vi "open close simple table.vi"(8 "error in (no error)":errorcluster) -> (0 "error out":errorcluster)   [LabVIEW 2020]
uses:
  forms AF/Autoclose manager/Form ID.ctl
  forms AF/Open Close Logic Simple Table/Open Close Logic Simple Table.lvclass
  <vilib>/addons/_JKI Toolkits/Caraya/classes/Assert/Assert Equal Value_Variant.vi
  forms AF/Form Server Interfaces.lvlib
  <vilib>/addons/_JKI Toolkits/Caraya/classes/Assert/Assert.lvclass
  <vilib>/addons/_JKI Toolkits/Caraya/classes/Test/Test.lvclass
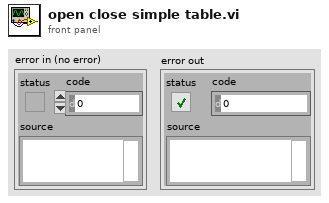
[diagram p1: front panel]
types:
  T1 = typedef "Form Server Interfaces.lvlib/Form ID.ctl" = cluster{"Name":string, "Panel type":string}
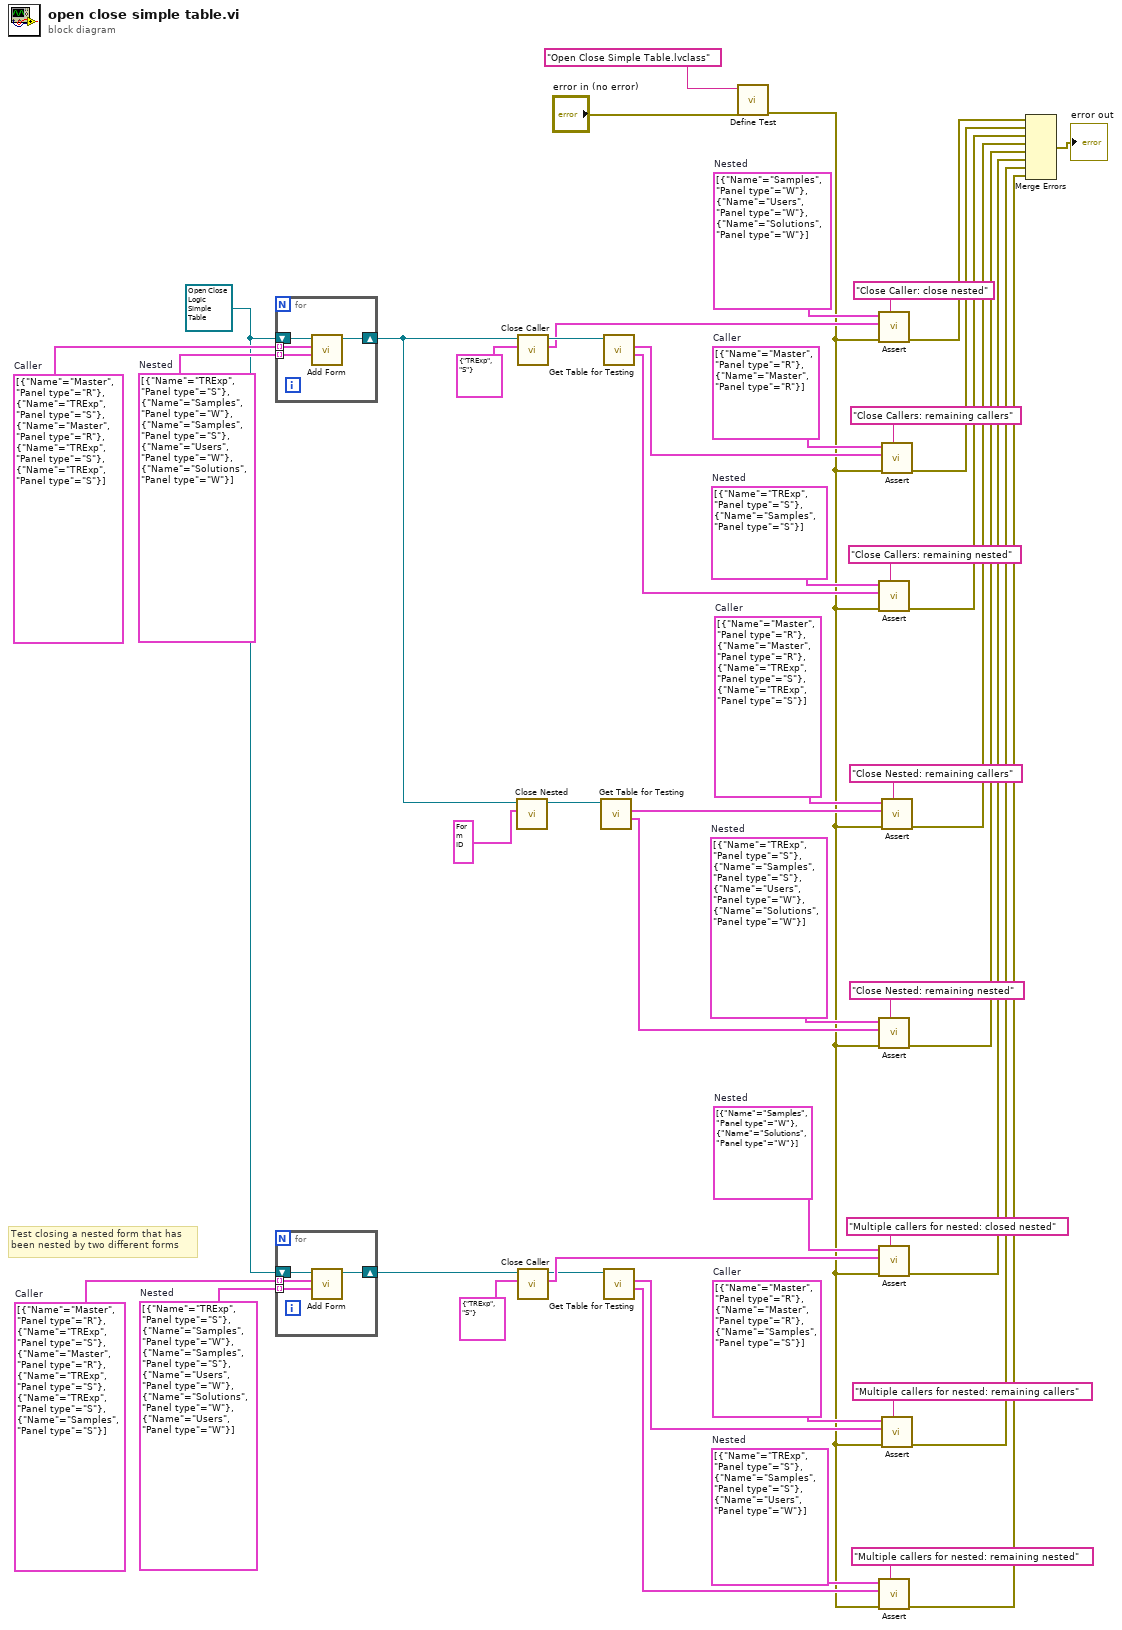
[diagram p0: block diagram]
diagram:
  w25 = T1[] [{"Name"="TRExp", "Panel type"="S"}, {"Name"="Samples", "Panel type"="S"}, {"Name"="Users", "Panel type"="W"}]  # Nested
  w21 = T1[] [{"Name"="Samples", "Panel type"="W"}, {"Name"="Solutions", "Panel type"="W"}]  # Nested
  w23 = T1[] [{"Name"="Master", "Panel type"="R"}, {"Name"="Master", "Panel type"="R"}, {"Name"="Samples", "Panel type"="S"}]  # Caller
  w31 = T1[] [{"Name"="TRExp", "Panel type"="S"}, {"Name"="Samples", "Panel type"="S"}, {"Name"="Users", "Panel type"="W"}, {"Name"="Solutions", "Panel type"="W"}]  # Nested
  w32 = T1[] [{"Name"="Master", "Panel type"="R"}, {"Name"="Master", "Panel type"="R"}, {"Name"="TRExp", "Panel type"="S"}, {"Name"="TRExp", "Panel type"="S"}]  # Caller
  w37 = T1[] [{"Name"="TRExp", "Panel type"="S"}, {"Name"="Samples", "Panel type"="S"}]  # Nested
  w41 = T1[] [{"Name"="Samples", "Panel type"="W"}, {"Name"="Users", "Panel type"="W"}, {"Name"="Solutions", "Panel type"="W"}]  # Nested
  w39 = T1[] [{"Name"="Master", "Panel type"="R"}, {"Name"="Master", "Panel type"="R"}]  # Caller
  w44 = T1[] [{"Name"="TRExp", "Panel type"="S"}, {"Name"="Samples", "Panel type"="W"}, {"Name"="Samples", "Panel type"="S"}, {"Name"="Users", "Panel type"="W"}, {"Name"="Solutions", "Panel type"="W"}, {"Name"="Users", "Panel type"="W"}]  # Nested
  w43 = T1[] [{"Name"="Master", "Panel type"="R"}, {"Name"="TRExp", "Panel type"="S"}, {"Name"="Master", "Panel type"="R"}, {"Name"="TRExp", "Panel type"="S"}, {"Name"="TRExp", "Panel type"="S"}, {"Name"="Samples", "Panel type"="S"}]  # Caller
  w26 = refnum<class "Open Close Logic Simple Table.lvclass"> refnum ("Open Close Logic Simple Table.lvlib:Open Close Logic Simple Table.lvclass")
  w48 = T1[] [{"Name"="TRExp", "Panel type"="S"}, {"Name"="Samples", "Panel type"="W"}, {"Name"="Samples", "Panel type"="S"}, {"Name"="Users", "Panel type"="W"}, {"Name"="Solutions", "Panel type"="W"}]  # Nested
  w49 = T1[] [{"Name"="Master", "Panel type"="R"}, {"Name"="TRExp", "Panel type"="S"}, {"Name"="Master", "Panel type"="R"}, {"Name"="TRExp", "Panel type"="S"}, {"Name"="TRExp", "Panel type"="S"}]  # Caller
  # "Test closing a nested form that has\nbeen nested by two different forms"
  n1 = for {
    tunnel: w49 -> [w51] mode=indexing
    tunnel: w48 -> [w50] mode=indexing
    shift-right: [w53] -> w47
    shift-left: w26 -> [w52]
    n2 = call-dynamic "Add Form.vi"("Nested"=w50, "Caller"=w51, "Autoclose manager in"=w52) -> ("Autoclose manager out"=w53:refnum<class "Open Close Logic Simple Table.lvclass">)  [unwired: 6 in, 2 out]
  }
  n3 = for {
    tunnel: w43 -> [w55] mode=indexing
    tunnel: w44 -> [w54] mode=indexing
    shift-right: [w57] -> w17
    shift-left: w26 -> [w56]
    n4 = call-dynamic "Add Form.vi"("Nested"=w54, "Caller"=w55, "Autoclose manager in"=w56) -> ("Autoclose manager out"=w57:refnum<class "Open Close Logic Simple Table.lvclass">)  [unwired: 6 in, 2 out]
  }
  n5 = call-dynamic "Close Nested.vi"("Nested"=T1 {"Name"="Samples", "Panel type"="W"}, "Open Close Logic Simple Table in"=w47) -> ("Open Close Logic Simple Table out"=w45:refnum<class "Open Close Logic Simple Table.lvclass">)  [unwired: 8 in, 1 out]
  n6 = call-dynamic "Close Caller.vi"("Caller"=T1 {"Name"="TRExp", "Panel type"="S"}, "Open Close Logic Simple Table in"=w47) -> ("Close Nested"=w42:T1[], "Open Close Logic Simple Table out"=w46:refnum<class "Open Close Logic Simple Table.lvclass">)  [unwired: 7 in, 1 out]
  n7 = call-dynamic "Close Caller.vi"("Caller"=T1 {"Name"="TRExp", "Panel type"="S"}, "Open Close Logic Simple Table in"=w17) -> ("Close Nested"=w20:T1[], "Open Close Logic Simple Table out"=w19:refnum<class "Open Close Logic Simple Table.lvclass">)  [unwired: 7 in, 1 out]
  n8 = call "Get Table for Testing.vi"("Open Close Logic Simple Table in"=w45) -> ("Nested"=w29:T1[], "Caller"=w30:T1[])  [unwired: 7 in, 2 out]
  n9 = call "Get Table for Testing.vi"("Open Close Logic Simple Table in"=w46) -> ("Nested"=w38:T1[], "Caller"=w40:T1[])  [unwired: 7 in, 2 out]
  n10 = call "Get Table for Testing.vi"("Open Close Logic Simple Table in"=w19) -> ("Nested"=w24:T1[], "Caller"=w22:T1[])  [unwired: 7 in, 2 out]
  n11 = call <vilib>:"Define Test.vi"("error in (no error)"="error in (no error)", "Label (VI Title)"="Open Close Simple Table.lvclass") -> ("error out"=w12:errorcluster)  [unwired: 9 in]
  n12 = call-poly <vilib>:"Assert.vi"("Label"="Close Caller: close nested", "error in (no error)"=w12, "Y"=w42, "X"=w41) -> ("error out"=w36:errorcluster)  [unwired: 7 in]
  n13 = call-poly <vilib>:"Assert.vi"("Label"="Close Callers: remaining nested", "error in (no error)"=w12, "Y"=w38, "X"=w37) -> ("error out"=w34:errorcluster)  [unwired: 7 in]
  n14 = call-poly <vilib>:"Assert.vi"("Label"="Close Nested: remaining nested", "error in (no error)"=w12, "Y"=w29, "X"=w31) -> ("error out"=w27:errorcluster)  [unwired: 7 in]
  n15 = call-poly <vilib>:"Assert.vi"("Label"="Multiple callers for nested: closed nested", "error in (no error)"=w12, "Y"=w20, "X"=w21) -> ("error out"=w15:errorcluster)  [unwired: 7 in]
  n16 = call-poly <vilib>:"Assert.vi"("Label"="Multiple callers for nested: remaining nested", "error in (no error)"=w12, "Y"=w24, "X"=w25) -> ("error out"=w7:errorcluster)  [unwired: 7 in]
  n17 = call-poly <vilib>:"Assert.vi"("Label"="Close Callers: remaining callers", "error in (no error)"=w12, "Y"=w40, "X"=w39) -> ("error out"=w35:errorcluster)  [unwired: 7 in]
  n18 = call-poly <vilib>:"Assert.vi"("Label"="Close Nested: remaining callers", "error in (no error)"=w12, "Y"=w30, "X"=w32) -> ("error out"=w28:errorcluster)  [unwired: 7 in]
  n19 = call-poly <vilib>:"Assert.vi"("Label"="Multiple callers for nested: remaining callers", "error in (no error)"=w12, "Y"=w22, "X"=w23) -> ("error out"=w14:errorcluster)  [unwired: 7 in]
  n20 = Merge Errors(w36, w35, w34, w28, w27, w15, w14, w7) -> (→"error out":errorcluster)
